vi "NewtonsPSM_StartStop.vi"(0 "VISA session":refnum<visa-resource-name>, 5 "Hold (F: ON)":bool=TRUE, 11 "error in (no error)":errorcluster) -> (4 "dup VISA session":refnum<visa-resource-name>, 15 "error out":errorcluster)   [LabVIEW 2025, in "NewtonsPSM1735.lvlib"]
doc: "This VI sends the Start or Stop Command for Integrator or Datalog Mode"
uses:
  NewtonsPSM1735.lvlib
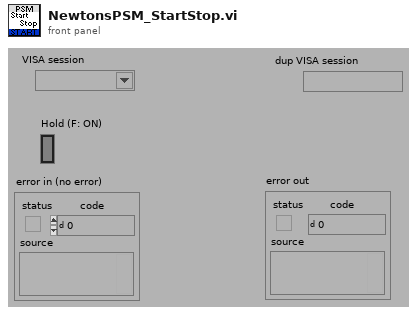
[diagram p1: front panel]
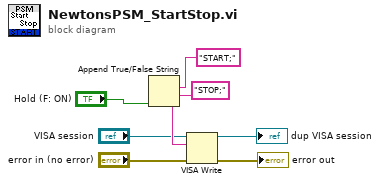
[diagram p0: block diagram]
diagram:
  n1 = Append True/False String(1:"Hold (F: ON)", 2:"STOP;", 3:"START;") -> (0:w8:string)  [unwired: 1 out]
  n2 = VISA Write(VISA resource name="VISA session", write buffer=w8, error in (no error)="error in (no error)") -> (VISA resource name out=→"dup VISA session":refnum<visa-resource-name>, error out=→"error out":errorcluster)  [unwired: 1 out]
